vi "Get ID.vi"(11 "IConnection in":refnum<class "IConnection.lvclass">) -> (2 "ID":string)   [LabVIEW 2019, in "Network Interface.lvlib" / "IConnection.lvclass"]
uses:
  <vilib>/gpm_packages/@cs/Network-Sink/Source/Network Interface/IConnection/IConnection.lvclass
  <vilib>/gpm_packages/@cs/Network-Sink/Source/Network Interface/IConnection/IConnection.lvclass/IConnection.ctl
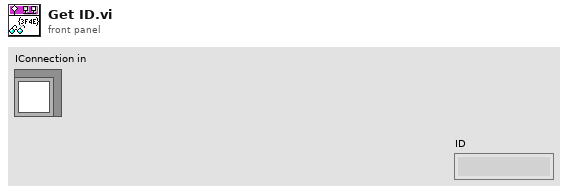
[diagram p1: front panel]
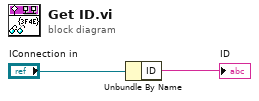
[diagram p0: block diagram]
diagram:
  n1 = Unbundle By Name("IConnection in") -> ("ID"=→"ID":string)
